vi "Ejercicio_3_Tabla_Indicador.vi"() -> ()   [LabVIEW 2020]
panel:
  out "Tabla Información":string[][](table)
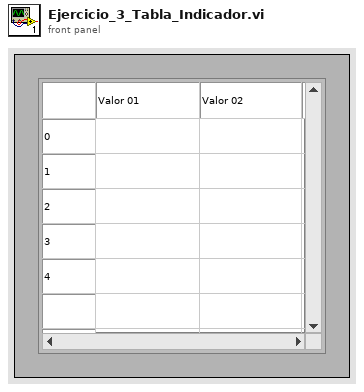
[diagram p1: front panel]
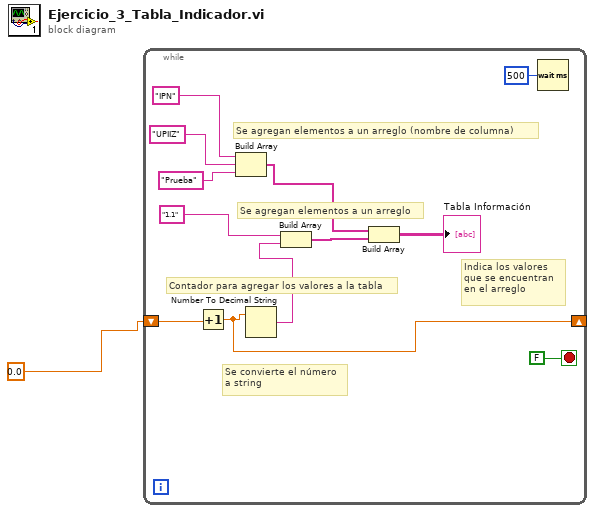
[diagram p0: block diagram]
diagram:
  n1 = while {
    shift-right: [w2] -> _
    shift-left: 0.0 -> [w4]
    stop <- FALSE stop-if-true
    # "Indica los valores\nque se encuentran \nen el arreglo"
    # "Se agregan elementos a un arreglo"
    # "Contador para agregar los valores a la tabla"
    # "Se agregan elementos a un arreglo (nombre de columna)"
    # "Se convierte el número\na string"
    n2 = Increment(x=w4) -> (x+1=w2:dbl)
    n3 = Build Array("IPN", "UPIIZ", "Prueba" ("element")) -> (w10:string[])
    n4 = Number To Decimal String(number=w2) -> (decimal integer string=w3:string)  [unwired: 1 in]
    n5 = Build Array("1.1", w3) -> (w8:string[])
    n6 = Build Array(w10, w8) -> (→"Tabla Información":string[][])
    n7 = Wait (ms)(milliseconds to wait=u32 500) -> ()  [unwired: 1 out]
  }
